vi "svl_Exponential Filter with IC.vi"(8 "init/cont (init:F)":bool, 9 "initial filter state":dbl format="%.2f", 10 "filter coefficients":T1 {"Forward Coefficients" format="%.2f"; "Reverse Coefficients" format="%.2f"}, 11 "X":dbl[](array[numeric]) format="%.2f") -> (0 "error":i32, 1 "final filter state":dbl format="%.2f", 3 "filtered X":dbl[](array[numeric]) format="%.2f")   [LabVIEW 2017]
doc: "Applies a single time constant exponential averaging on the input signal X based on the filter coefficients and returns the entire filtered signal.\nThe initial filter state and the final filter state parameters keep track of the internal state of the filter to ensure continuous operation of the filter if continuous mode is used."
uses:
  <vilib>/Analysis/NI_AALBase.lvlib
panel:
  # "Exponential Filter with I.C."
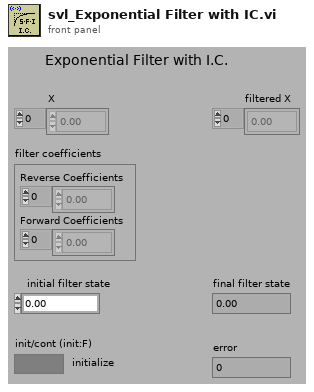
[diagram p1: front panel]
types:
  T1 = cluster{"Reverse Coefficients":dbl[], "Forward Coefficients":dbl[]}
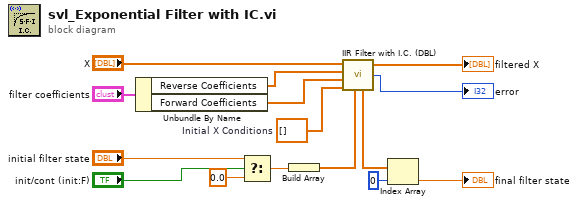
[diagram p0: block diagram]
diagram:
  w6 = dbl[] []  # Initial X Conditions
  n1 = Unbundle By Name("filter coefficients") -> ("Reverse Coefficients"=w10:dbl[], "Forward Coefficients"=w9:dbl[])
  n2 = Select(t="initial filter state", s="init/cont (init:F)", f=0.0) -> (s? t:f=w1:dbl)
  n3 = Build Array(w1) -> (w5:dbl[])
  n4 = call <vilib>:"IIR Filter with I.C. (DBL).vi"("Initial Y Conditions"=w5, "Initial X Conditions"=w6, "Forward Coefficients"=w9, "Reverse Coefficients"=w10, "X"="X") -> ("Final Y Conditions"=w7:dbl[], "error"=→"error":i32, "Filtered X"=→"filtered X":dbl[])  [unwired: 2 in, 1 out]
  n5 = Index Array(array=w7, index=0) -> (element=→"final filter state":dbl)
